vi "Timestamp2DayofYear.vi"(7 "time stamp":timestamp) -> (8 "time string":string)   [LabVIEW 2019]
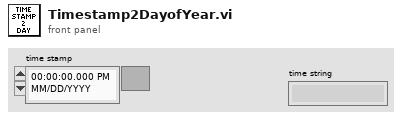
[diagram p1: front panel]
types:
  T1 = typedef "LVDateTimeRec.ctl" = cluster{"fractional second":dbl, "second":i32, "minute":i32, "hour":i32, "day of month":i32, "month":i32, "year":i32, "day of week":i32, "day of year":i32, "DST":i32}
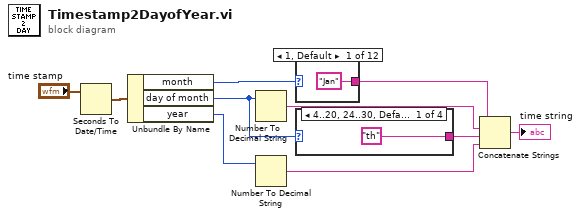
[diagram p0: block diagram]
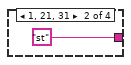
[diagram p2: hidden frame]
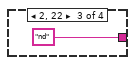
[diagram p3: hidden frame]
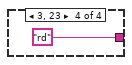
[diagram p4: hidden frame]
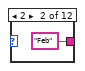
[diagram p5: hidden frame]
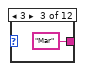
[diagram p6: hidden frame]
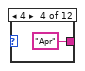
[diagram p7: hidden frame]
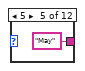
[diagram p8: hidden frame]
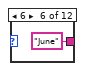
[diagram p9: hidden frame]
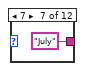
[diagram p10: hidden frame]
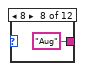
[diagram p11: hidden frame]
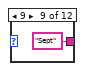
[diagram p12: hidden frame]
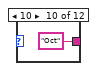
[diagram p13: hidden frame]
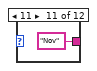
[diagram p14: hidden frame]
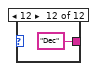
[diagram p15: hidden frame]
diagram:
  n1 = Seconds To Date/Time(time stamp (now)="time stamp") -> (date time rec=w4:T1)  [unwired: 1 in]
  n2 = Unbundle By Name(w4) -> ("month"=w5:i32, "day of month"=w1:i32, "year"=w9:i32)
  n3 = Number To Decimal String(number=w1) -> (decimal integer string=w6:string)  [unwired: 1 in]
  n4 = Number To Decimal String(number=w9) -> (decimal integer string=w10:string)  [unwired: 1 in]
  n5 = case shown="1, Default" w5 {
    tunnel: ["Jan" "Feb" "Mar" "Apr" "May" "June" "July" "Aug" "Sept" "Oct" "Nov" "Dec"] -> w8
    frame 1, Default {
    }
    frame 2 {
    }
    frame 3 {
    }
    frame 4 {
    }
    frame 5 {
    }
    frame 6 {
    }
    frame 7 {
    }
    frame 8 {
    }
    frame 9 {
    }
    frame 10 {
    }
    frame 11 {
    }
    frame 12 {
    }
  }
  n6 = case shown="4..20, 24..30, Default" w1 {
    tunnel: ["th" "st" "nd" "rd"] -> w7
    frame 4..20, 24..30, Default {
    }
    frame 1, 21, 31 {
    }
    frame 2, 22 {
    }
    frame 3, 23 {
    }
  }
  n7 = Concatenate Strings(w8, w6, w7, w10) -> (→"time string":string)
